vi "Capture_RGB_20Fibers.vi"() -> ()   [LabVIEW 2018]
panel:
  in  "Capture Range":u32(ring) items=["Auto", "Low", "Medium", "High", "Super", "Ultra"]
  in  "isPWM":bool
  in  "VISA resource name":refnum<visa-resource-name>="ASRL34::INSTR"
  out "Table":string[][](table)
  # "NOTE: remember plug the LED Analyser\nbefore run this VI and to change the\nVISA resource name (port) in the panel,\notherwise the application will not work."
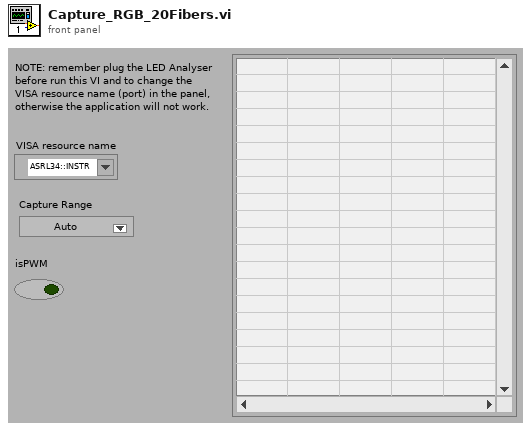
[diagram p1: front panel]
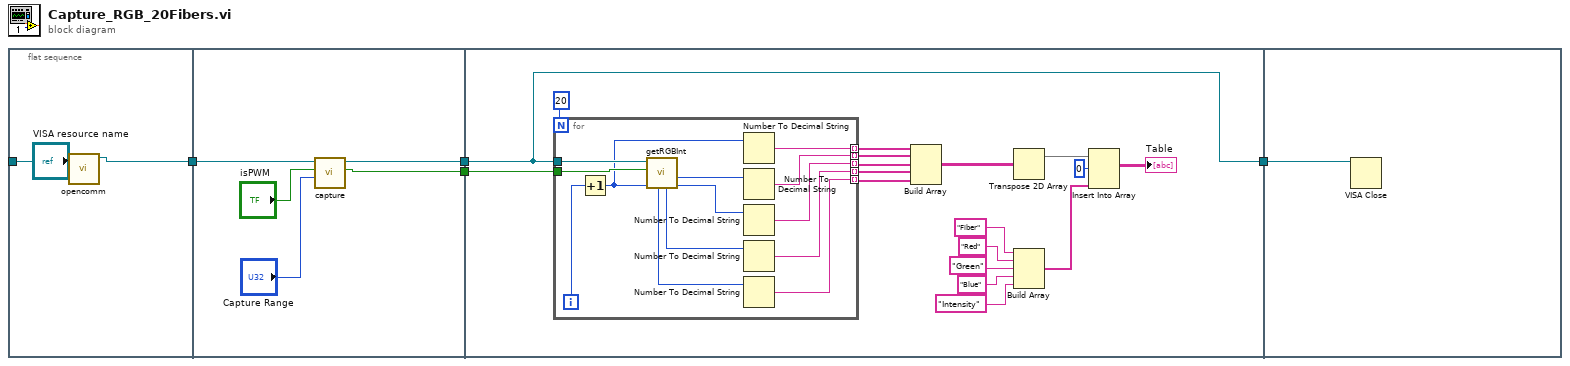
[diagram p0: block diagram]
diagram:
  n1 = flat-sequence {
    tunnel: "VISA resource name" -> [w7]
    tunnel: [w6] -> w4
    tunnel: w4 -> [w12]
    tunnel: [w11] -> w3
    tunnel: [w8] -> w1
    tunnel: w3 -> [w30]
    tunnel: [w30] -> w2
    tunnel: w1 -> [w13]
    tunnel: w2 -> [w44]
    frame #0 {
      n2 = call "opencomm.vi"("VISA resource name"=w7) -> ("duplicate VISA resource name"=w6:refnum<visa-resource-name>)  [unwired: 3 in, 1 out]
    }
    frame #1 {
      n3 = call "capture.vi"("Capture Range (0, auto)"="Capture Range", "isPWM (no)"="isPWM", "VISA resource name"=w12) -> ("Error"=w8:bool, "dup VISA resource name"=w11:refnum<visa-resource-name>)  [unwired: 3 in]
    }
    frame #2 {
      n4 = for {
        N: 20 -> [_]
        tunnel: w30 -> [w41]
        tunnel: [w34] -> w28 mode=indexing
        tunnel: [w33] -> w27 mode=indexing
        tunnel: [w32] -> w26 mode=indexing
        tunnel: [w31] -> w25 mode=indexing
        tunnel: [w43] -> w23 mode=indexing
        tunnel: w13 -> [w40]
        i -> [w42]
        n5 = Increment(x=w42) -> (x+1=w39:i32)
        n6 = call "getRGBInt.vi"("Fiber Num"=w39, "Error"=w40, "VISA resource name"=w41) -> ("Green"=w38:u8, "Red"=w37:u8, "Blue"=w36:u8, "Intensity"=w35:u32)  [unwired: 3 in, 2 out]
        n7 = Number To Decimal String(number=w39) -> (decimal integer string=w43:string)  [unwired: 1 in]
        n8 = Number To Decimal String(number=w37) -> (decimal integer string=w34:string)  [unwired: 1 in]
        n9 = Number To Decimal String(number=w38) -> (decimal integer string=w33:string)  [unwired: 1 in]
        n10 = Number To Decimal String(number=w36) -> (decimal integer string=w32:string)  [unwired: 1 in]
        n11 = Number To Decimal String(number=w35) -> (decimal integer string=w31:string)  [unwired: 1 in]
      }
      n12 = Build Array(w23, w28, w27, w26, w25) -> (w24:string[][])
      n13 = Transpose 2D Array(2D array=w24) -> (transposed array=w21:string[][])
      n14 = Build Array("Fiber", "Red", "Green", "Blue", "Intensity") -> (w15:string[])
      n15 = Insert Into Array(array=w21, index (row)=0 ("Index (row)"), new element=w15) -> (→"Table":string[][])  [unwired: 1 in]
    }
    frame #3 {
      n16 = VISA Close(VISA resource name=w44) -> ()  [unwired: 1 in, 1 out]
    }
  }
